vi "公式输入子VI .vi"() -> (0 "生成的波形":waveform(dbl)(graph), 1 "最小值":dbl format="%#_3g", 2 "最大值":dbl format="%#_3g")   [LabVIEW 2017]
uses:
  <vilib>/measure/NI_MAPro.lvlib
panel:
  in  "样本数":dbl=1000.0
  in  "采样率":dbl=1000.0
  in  "频率":dbl=10.0
  in  "公式":string="sin(w*t)*sin(2*pi(1)*t)"
  in  "完成":bool
  # "公式 输 入"
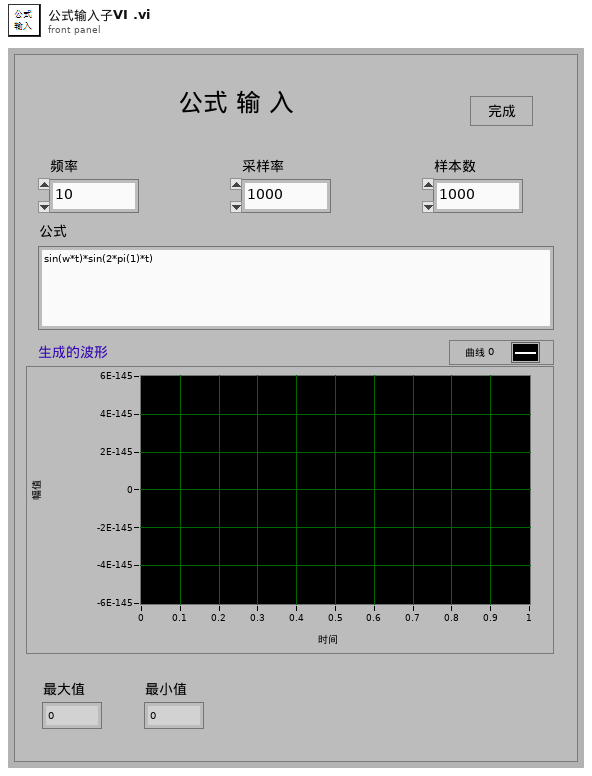
[diagram p1: front panel]
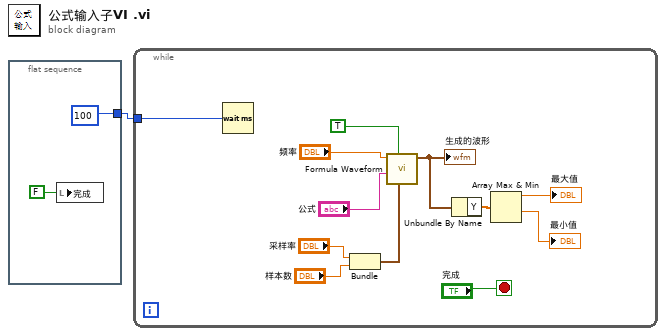
[diagram p0: block diagram]
diagram:
  n1 = flat-sequence {
    tunnel: [u32 100 ("等待时间（毫秒）")] -> w1
    frame #0 {
      n2 = local write "完成"(FALSE ("完成")) -> ()
    }
  }
  n3 = while {
    tunnel: w1 -> [w5]
    stop <- "完成" stop-if-true
    n4 = Wait (ms)(milliseconds to wait=w5) -> ()  [unwired: 1 out]
    n5 = Bundle("采样率"="采样率", "样本数"="样本数") -> (w6:cluster{"采样率":dbl, "样本数":dbl})  [unwired: 1 in]
    n6 = call <vilib>:"Formula Waveform.vi"("sampling info"=w6, "reset signal"=TRUE, "formula"="公式", "frequency"="频率") -> ("signal out"=w9:waveform(dbl))  [unwired: 6 in, 1 out]
    "生成的波形" <- w9
    n7 = Unbundle By Name(w9) -> ("Y"=w14:dbl[])
    n8 = Array Max & Min(array=w14) -> (max value=→"最大值":dbl, min value=→"最小值":dbl)  [unwired: 2 out]
  }
